vi "ADC_get_array.vi"(5 "Inst_parameter":T1) -> (0 "Readout error":bool, 1 "measures":sgl[][](array[numeric]), 2 "Inst_parameter out":T1)   [LabVIEW 2013]
uses:
  <vilib>/DAQmx/read.llb/DAQmx Read (Analog 2D DBL NChan NSamp).vi
  <vilib>/Analysis/baseanly.llb/Mean (DBL).vi
  <vilib>/DAQmx/miscellaneous.llb/DAQmx Fill In Error Info.vi
  <resource>/objmgr/daqmx.rc
  <vilib>/Analysis/NI_AALBase.lvlib
panel:
  in  "Emergency stop":bool
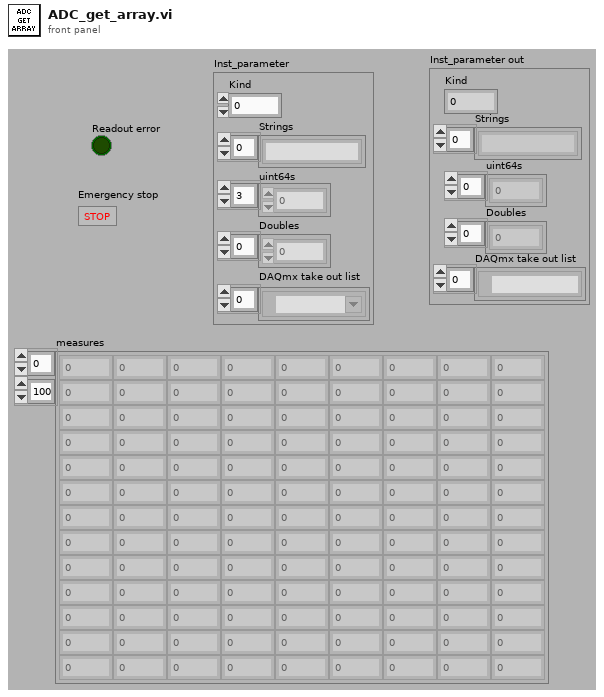
[diagram p1: front panel]
types:
  T1 = cluster{"Kind":u16, "Strings":string[], "uint64s":u64[], "Doubles":dbl[], "DAQmx take out list":refnum<k21>[]}
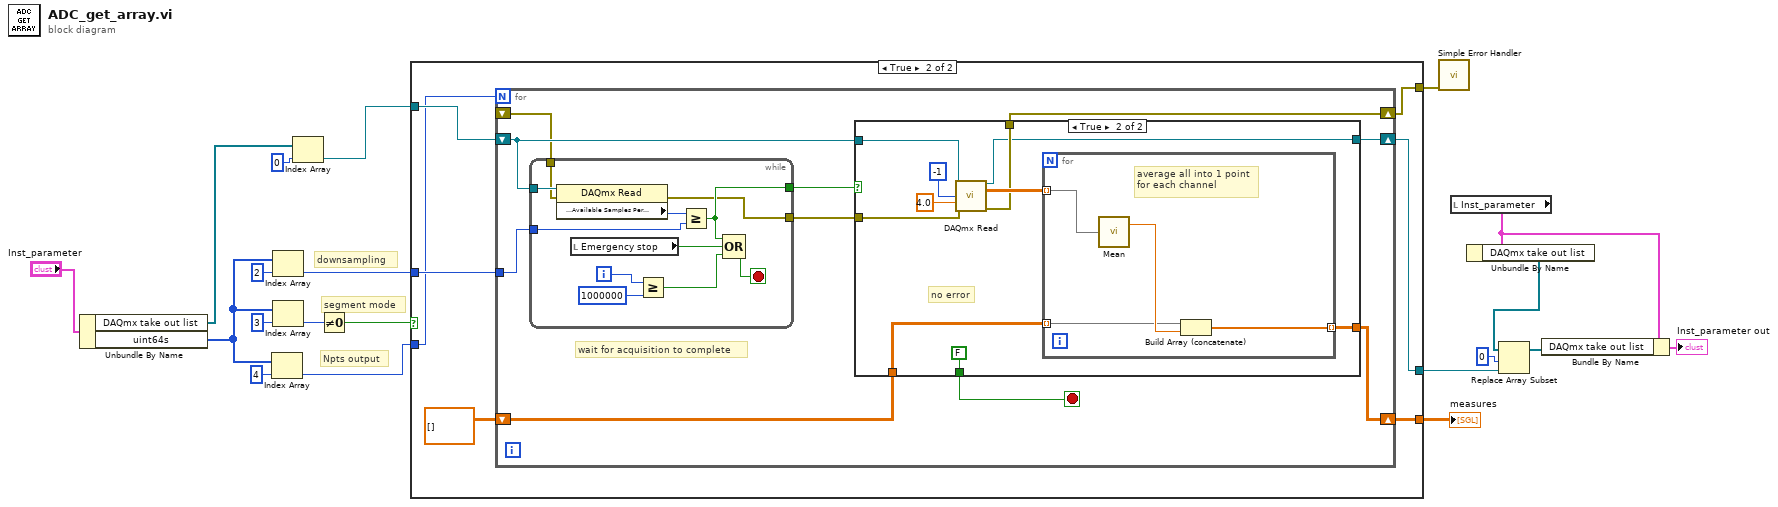
[diagram p0: block diagram]
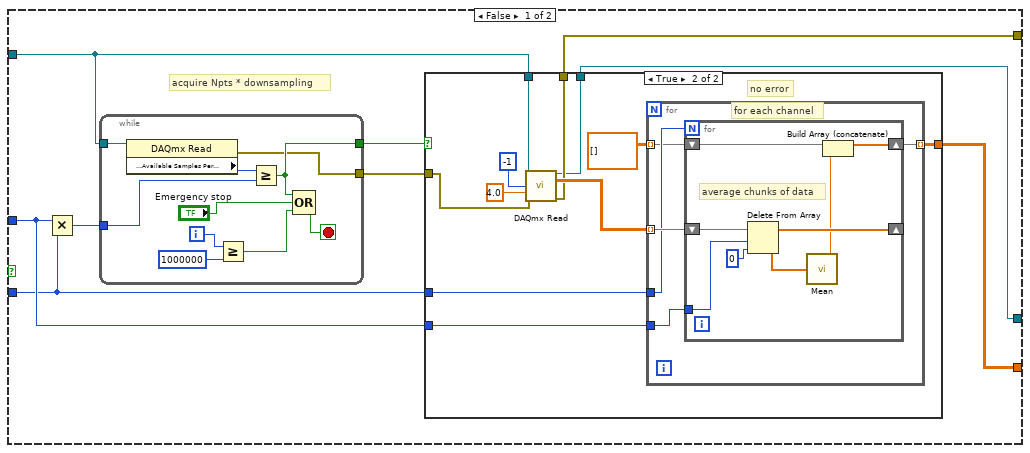
[diagram p2: hidden frame]
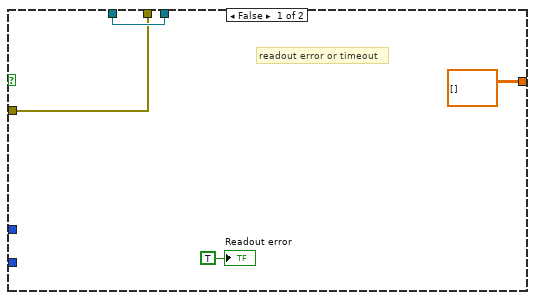
[diagram p3: hidden frame]
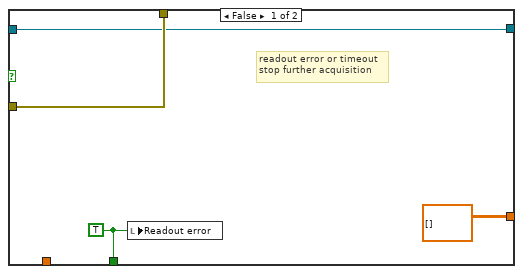
[diagram p4: hidden frame]
diagram:
  # "Npts output"
  # "segment mode"
  # "downsampling"
  n1 = Unbundle By Name("Inst_parameter") -> ("DAQmx take out list"=w10:refnum<k21>[], "uint64s"=w14:u64[])
  n2 = Index Array(array=w14, index=4) -> (element=w6:u64)
  n3 = Index Array(array=w14, index=2) -> (element=w11:u64)
  n4 = Index Array(array=w14, index=3) -> (element=w13:u64)
  n5 = Index Array(array=w10, index=0) -> (element=w9:refnum<k21>)
  n6 = Not Equal To 0?(x=w13) -> (x != 0?=w12:bool)
  n7 = case shown="True" w12 {
    tunnel: w11 -> [w26 w73]
    tunnel: w9 -> [w21 w74]
    tunnel: [w23 w71] -> w1
    tunnel: [w25 w70] -> w7
    tunnel: w6 -> [w24 w69]
    tunnel: [w22 w68] -> w5
    frame False {
      # "acquire Npts * downsampling"
      n8 = Multiply(x=w26, y=w24) -> (x*y=w29:u64)
      n9 = while {
        tunnel: w21 -> [w67]
        tunnel: w29 -> [w62]
        tunnel: [w64] -> w28
        tunnel: [w63] -> w27
        i -> [w61]
        stop <- w65 stop-if-true
        n10 = property class="DAQmx Read"(reference=w67) -> (error out=w63:errorcluster, "Status:Available Samples Per Channel"=w66:u32)  [unwired: 1 in, 1 out]
        n11 = Greater Or Equal?(x=w61, y=1000000) -> (x >= y?=w58:bool)
        n12 = Greater Or Equal?(x=w66, y=w62) -> (x >= y?=w64:bool)
        n13 = Compound Arithmetic op=OR(w64, "Emergency stop", w58) -> (w65:bool)
      }
      n14 = case shown="True" w28 {
        tunnel: w21 -> [w31 w42]
        tunnel: w27 -> [w30 w41]
        tunnel: w24 -> [_ w39]
        tunnel: w26 -> [_ w38]
        tunnel: [dbl[][] [] ("data") w36] -> w23
        tunnel: [w30 w35] -> w25
        tunnel: [w31 w34] -> w22
        frame False {
          # "readout error or timeout"
          "Readout error" <- TRUE ("Readout error")
        }
        frame True {
          # "no error"
          n15 = call-poly <vilib>:"DAQmx Read.vi"("task/channels in"=w42, "number of samples per channel"=-1, "timeout"=4.0, "error in"=w41) -> ("task out"=w34:refnum<k21>, "data"=w40:dbl[][], "error out"=w35:errorcluster)  [unwired: 9 out]
          n16 = for {
            tunnel: w38 -> [w48]
            tunnel: w39 -> [w47]
            tunnel: w40 -> [w49] mode=indexing
            tunnel: dbl[][] [] ("data") -> [w46] mode=indexing
            tunnel: [w45] -> w36 mode=indexing
            # "for each channel"
            n17 = for {
              N: w47 -> [_]
              shift-right: [w55] -> _
              shift-left: w49 -> [w57]
              tunnel: w48 -> [w56]
              shift-right: [w51] -> w45
              shift-left: w46 -> [w52]
              # "average chunks of data"
              n18 = Delete From Array(array=w57, length=w56, index=0) -> (deleted portion=w53:dbl[], array with subset deleted=w55:dbl[])
              n19 = call-poly <vilib>:"Mean.vi"("X"=w53) -> ("mean"=w50:dbl)  [unwired: 1 out]
              n20 = Build Array (concatenate)(w52, w50) -> (w51:dbl[])
            }
          }
        }
      }
    }
    frame True {
      n21 = for {
        N: w69 -> [_]
        tunnel: w73 -> [w81]
        shift-right: [w79] -> w71
        shift-left: dbl[][] [] ("data") -> [w80]
        shift-right: [w77] -> w70
        shift-left: _ -> [w76]
        shift-right: [w75] -> w68
        shift-left: w74 -> [w83]
        stop <- w78 stop-if-true
        # "wait for acquisition to complete"
        n22 = while {
          tunnel: w83 -> [w113]
          tunnel: w81 -> [w111]
          tunnel: [w108] -> w84
          tunnel: [w107] -> w82
          tunnel: w76 -> [w106]
          i -> [w104]
          stop <- w109 stop-if-true
          n23 = property class="DAQmx Read"(reference=w113, error in=w106) -> (error out=w107:errorcluster, "Status:Available Samples Per Channel"=w112:u32)  [unwired: 1 out]
          n24 = local read "Emergency stop"() -> (w110:bool)
          n25 = Greater Or Equal?(x=w104, y=1000000) -> (x >= y?=w103:bool)
          n26 = Greater Or Equal?(x=w112, y=w111) -> (x >= y?=w108:bool)
          n27 = Compound Arithmetic op=OR(w108, w110, w103) -> (w109:bool)
        }
        n28 = case shown="True" w84 {
          tunnel: w83 -> [w85 w96]
          tunnel: w82 -> [w86 w95]
          tunnel: [dbl[][] [] ("data") w93] -> w79
          tunnel: w80 -> [_ w92]
          tunnel: [w87 FALSE ("Readout error")] -> w78
          tunnel: [w86 w90] -> w77
          tunnel: [w85 w89] -> w75
          frame False {
            w87 = TRUE ("Readout error")
            # "readout error or timeout\nstop further acquisition"
            n29 = local write "Readout error"(w87) -> ()
          }
          frame True {
            # "no error"
            n30 = call-poly <vilib>:"DAQmx Read.vi"("task/channels in"=w96, "number of samples per channel"=-1, "timeout"=4.0, "error in"=w95) -> ("task out"=w89:refnum<k21>, "data"=w94:dbl[][], "error out"=w90:errorcluster)  [unwired: 9 out]
            n31 = for {
              tunnel: w94 -> [w100] mode=indexing
              tunnel: [w102] -> w93 mode=indexing
              tunnel: w92 -> [w99] mode=indexing
              # "average all into 1 point\nfor each channel"
              n32 = call-poly <vilib>:"Mean.vi"("X"=w100) -> ("mean"=w101:dbl)  [unwired: 1 out]
              n33 = Build Array (concatenate)(w99, w101) -> (w102:dbl[])
            }
          }
        }
      }
    }
  }
  "measures" <- w1
  n34 = call <vilib>:"Simple Error Handler.vi"("error in (no error)"=w7) -> ()  [unwired: 4 in, 5 out]
  n35 = local read "Inst_parameter"() -> (w3:T1)
  n36 = Unbundle By Name(w3) -> ("DAQmx take out list"=w4:refnum<k21>[])
  n37 = Replace Array Subset(array=w4, new element=w5, index=0) -> (w20:refnum<k21>[])
  n38 = Bundle By Name(cluster=w3, "DAQmx take out list"=w20) -> (→"Inst_parameter out":T1)
